vi "TCP Close Server.vi"(8 "error in (no error)":errorcluster, 11 "SLL Easy API via TCP in":refnum<class "SLL Easy API via TCP.lvclass">) -> (0 "error out":errorcluster)   [LabVIEW 2014, in "SLL Easy API via TCP.lvclass"]
uses:
  SLL Easy API via TCP.lvclass
  SLL Easy API via TCP.lvclass/SLL Easy API via TCP.ctl
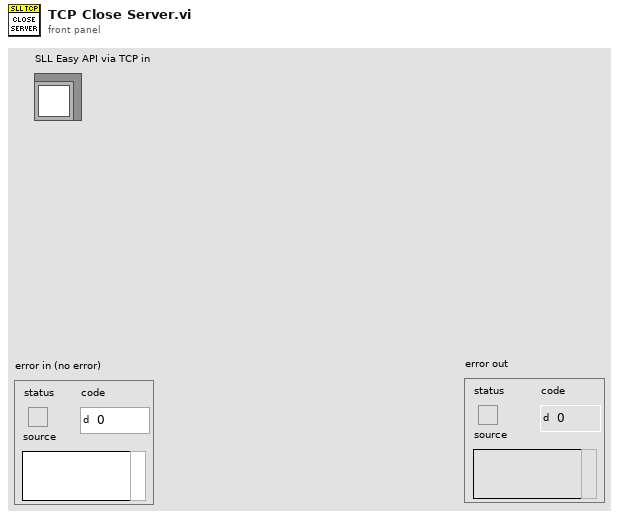
[diagram p1: front panel]
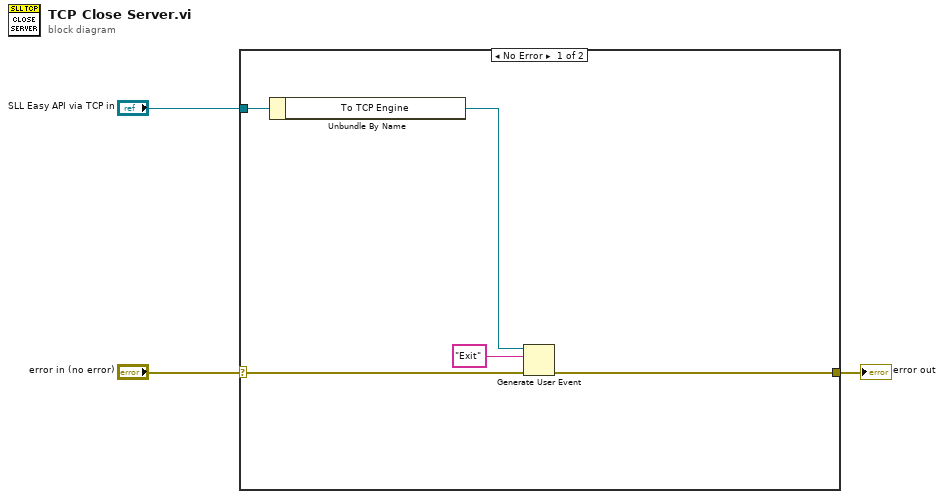
[diagram p0: block diagram]
diagram:
  n1 = case shown="No Error" "error in (no error)" {
    selector: "error in (no error)" -> [w7 w9]
    tunnel: [w6 w9] -> w2
    tunnel: "SLL Easy API via TCP in" -> [w8 _]
    frame No Error {
      n2 = Unbundle By Name(w8) -> ("To TCP Engine"=w5:refnum<user-event>)
      n3 = Generate User Event(user event=w5, event data cluster="Exit" ("event data"), error in=w7) -> (error out=w6:errorcluster)  [unwired: 1 in, 1 out]
    }
    frame Error {
    }
  }
  "error out" <- w2
